vi "RT Main.vi"() -> ()   [LabVIEW 2019]
doc: "Sends signals to the myRIO depending on what is received through UDP communication"
uses:
  <vilib>/myRIO/Common/Instrument Driver Framework/myRIO v1.0/UART/vis/myRIO v1.0 Close UART.vi
  <vilib>/myRIO/Common/Instrument Driver Framework/Utilities/vis/FPGA Ref Manager.vi
  <vilib>/myRIO/Common/Instrument Driver Framework/myRIO v1.0/myRIO v1.0 Reset FPGA.vi
  <vilib>/myRIO/Common/Instrument Driver Framework/myRIO v1.0/IRQ/vis/myRIO v1.0 IRQ Info FGV.vi
  <vilib>/myRIO/Common/Instrument Driver Framework/myRIO v1.0/IRQ/vis/myRIO v1.0 Timer IRQ Info FGV.vi
  <vilib>/myRIO/Common/Instrument Driver Framework/myRIO v1.0/IRQ/vis/myRIO v1.0 ISR Agent.vi
  <vilib>/myRIO/Instrument Drivers/Utilities/vis/Reset Index.vi
  <vilib>/myRIO/Common/Instrument Driver Framework/myRIO v1.0/Resource Manager/vis/myRIO v1.0 Block Write Resource Manager.vi
  <vilib>/myRIO/Instrument Drivers/Utilities/Utilities.lvlib
panel:
  in  "Stop":bool
  out "Cmd to Execute":string[](array[string])
  out "Lettre a execute":string
  out "error out":errorcluster
  # "Overview: Resolve a Rubik's cube or send some commands using User Datagram Protocol (UDP). \n\nInstructions:\n1. Run this VI.\n2. Open Desktop Main.vi and follow its front panel instructions.\n3. Click Stop to stop this VI."
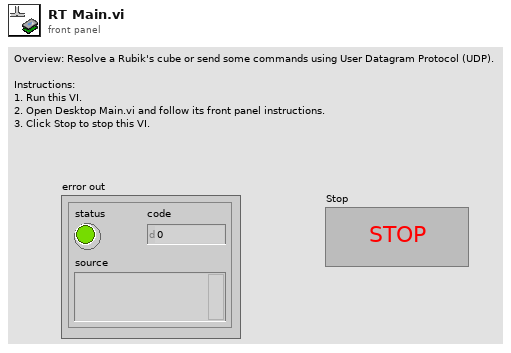
[diagram p1: front panel]
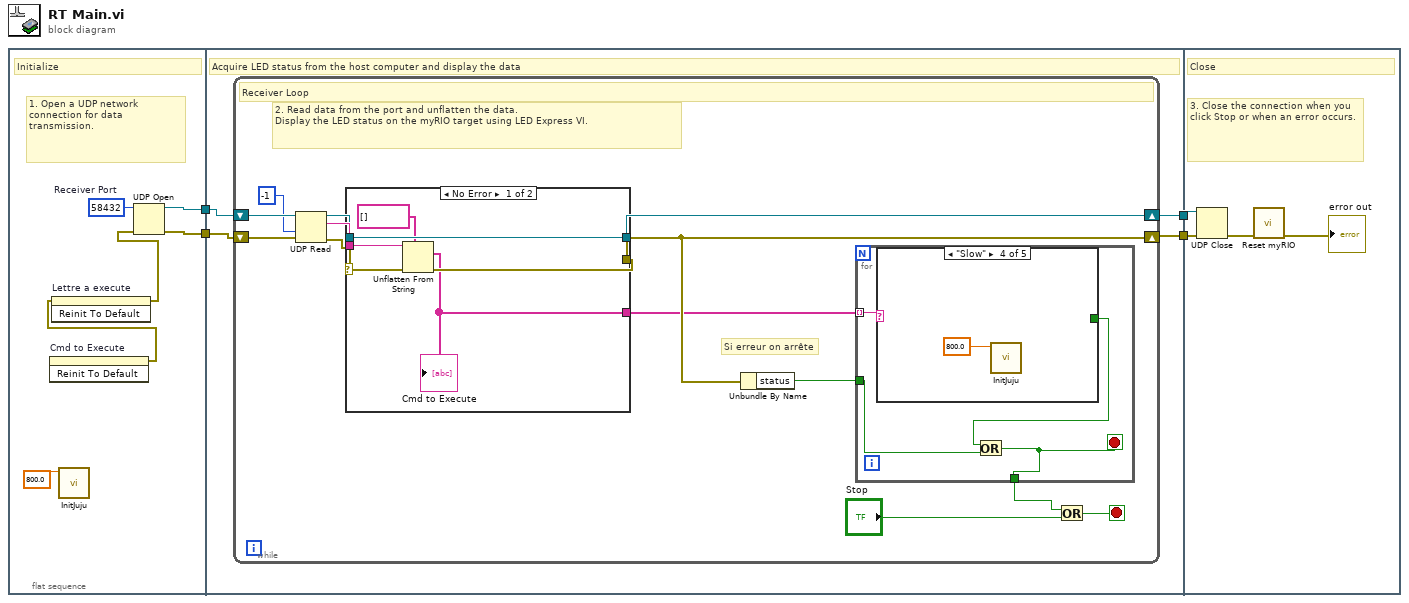
[diagram p0: block diagram]
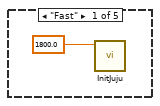
[diagram p2: hidden frame]
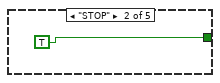
[diagram p3: hidden frame]
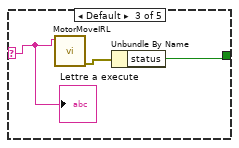
[diagram p4: hidden frame]
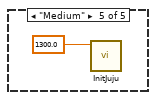
[diagram p5: hidden frame]
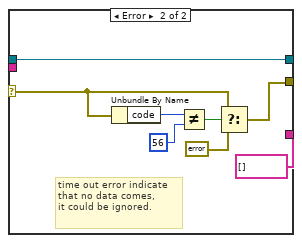
[diagram p6: hidden frame]
diagram:
  n1 = flat-sequence {
    tunnel: [w9] -> w4
    tunnel: [w8] -> w3
    tunnel: w4 -> [w12]
    tunnel: w3 -> [w11]
    tunnel: [w14] -> w2
    tunnel: [w13] -> w1
    tunnel: w2 -> [w54]
    tunnel: w1 -> [w53]
    frame #0 {
      w10 = u16 58432  # Receiver Port
      # "1. Open a UDP network connection for data transmission."
      # "Initialize"
      n2 = invoke on="Cmd to Execute" class="Arr (strict)" method="Reinit To Default"() -> (error out=w6:errorcluster)  [unwired: 3 in, 2 out]
      n3 = invoke on="Lettre a execute" class="Str" method="Reinit To Default"(error in=w6) -> (error out=w7:errorcluster)  [unwired: 2 in, 2 out]
      n4 = call "InitJuju.vi"("Frequency [Hz]"=800.0) -> ()  [unwired: 10 in, 1 out]
      n5 = UDP Open(8:w7, 11:w10) -> (port=w9:refnum<k16>, 0:w8:errorcluster)  [unwired: 3 in, 1 out]
    }
    frame #1 {
      # "Acquire LED status from the host computer and display the data"
      n6 = while {
        shift-right: [w20] -> w13
        shift-left: w11 -> [w26]
        shift-right: [w21] -> w14
        shift-left: w12 -> [w27]
        stop <- w17 stop-if-true
        # "Si erreur on arrête"
        # "2. Read data from the port and unflatten the data.\nDisplay the LED status on the myRIO target using LED Express VI."
        # "Receiver Loop"
        n7 = UDP Read(connection ID=w27, timeout ms (25000)=-1, 8:w26) -> (data out=w25:string, error out=w23:errorcluster, 3:w22:refnum<k16>)  [unwired: 1 in, 2 out]
        n8 = case shown="No Error" w23 {
          selector: w23 -> [w43 w47]
          tunnel: [w41 w46] -> w20
          tunnel: w25 -> [w44 _]
          tunnel: w22 -> [w42 w52]
          tunnel: [w42 w52] -> w21
          tunnel: [w39 string[] []] -> w15
          frame No Error {
            n9 = Unflatten From String(type=string[] [], binary string=w44, error in (no error)=w43) -> (value=w39:string[], error out=w41:errorcluster)  [unwired: 2 in, 1 out]
            "Cmd to Execute" <- w39
          }
          frame Error {
            # "time out error indicate that no data comes,\nit could be ignored."
            n10 = Unbundle By Name(w47) -> ("code"=w49:i32)
            n11 = Not Equal?(x=w49, y=56) -> (x != y?=w48:bool)
            n12 = Select(t=w47, s=w48, f=errorcluster {"status"=FALSE, "code"=0, "source"=""} ("error out")) -> (s? t:f=w46:errorcluster)
          }
        }
        n13 = Unbundle By Name(w20) -> ("status"=w19:bool)
        n14 = for {
          tunnel: w15 -> [w31] mode=indexing
          tunnel: [w28] -> w18
          tunnel: w19 -> [w29]
          stop <- w28 stop-if-true
          n15 = case shown="\"Slow\"" w31 {
            selector: w31 -> [_ _ w36 _ _]
            tunnel: [_ TRUE w34 _ _] -> w30
            frame "Fast" {
              n16 = call "InitJuju.vi"("Frequency [Hz]"=1800.0) -> ()  [unwired: 10 in, 1 out]
            }
            frame "STOP" {
            }
            frame Default {
              n17 = call "MotorMoveIRL.vi"("Rbt Cmd"=w36) -> ("error out"=w35:errorcluster)  [unwired: 10 in]
              n18 = Unbundle By Name(w35) -> ("status"=w34:bool)
              "Lettre a execute" <- w36
            }
            frame "Slow" {
              n19 = call "InitJuju.vi"("Frequency [Hz]"=800.0) -> ()  [unwired: 10 in, 1 out]
            }
            frame "Medium" {
              n20 = call "InitJuju.vi"("Frequency [Hz]"=1300.0) -> ()  [unwired: 10 in, 1 out]
            }
          }
          n21 = Or(x=w30, y=w29) -> (x .or. y?=w28:bool)
        }
        n22 = Or(x=w18, y="Stop") -> (x .or. y?=w17:bool)
      }
    }
    frame #2 {
      # "3. Close the connection when you click Stop or when an error occurs."
      # "Close"
      n23 = UDP Close(connection ID=w54, 8:w53) -> (error out=w56:errorcluster)  [unwired: 1 out]
      n24 = call <vilib>:"Reset myRIO.vi"("error in (no error)"=w56) -> ("error out"=→"error out":errorcluster)  [unwired: 10 in]
    }
  }
